vi "Download_All_(Single).vi"(7 "File Selection":i32, 8 "error in (no error)":errorcluster, 10 "Data":T1={"Info Box"="", "MAC & Name Out"=[], "Default Gateway"="", "Drfiter IP Addresses"=[], "Network Map"="", "Drifter Selection"=0, "File Selection"=0, "Download File Path"=path "", "File Selection Strings"=[], "Sample Rate"=enum." 0.2", "Log While Charging"=enum." Yes"}, 11 "File Path Control":path) -> (0 "error out":errorcluster)   [LabVIEW 2017]
uses:
  data.ctl
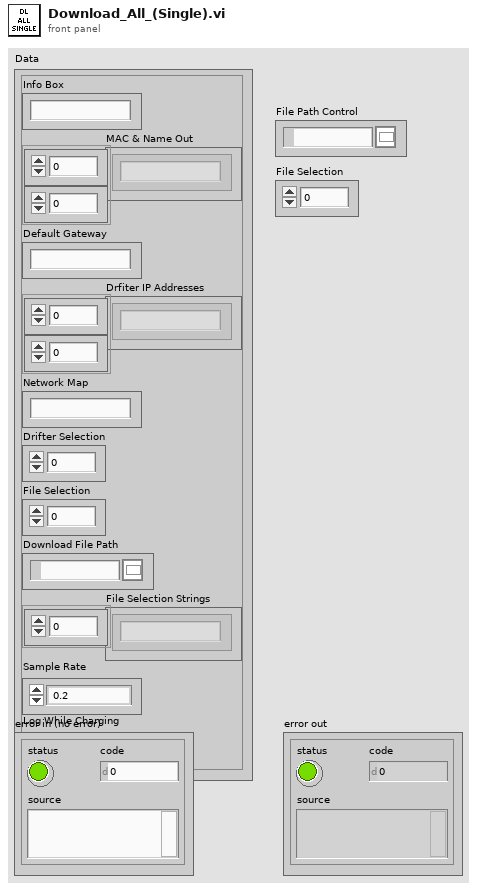
[diagram p1: front panel]
types:
  T1 = typedef "data.ctl" = cluster{"Info Box":string, "MAC & Name Out":string[][], "Default Gateway":string, "Drfiter IP Addresses":string[][], "Network Map":string, "Drifter Selection":i32, "File Selection":i32, "Download File Path":path, "File Selection Strings":string[], "Sample Rate":enum32{"No Selection", " 0.2", " 0.1", " 1", " 2", " 5", " 10"}, "Log While Charging":enum32{"No Selection", " Yes", " No"}}
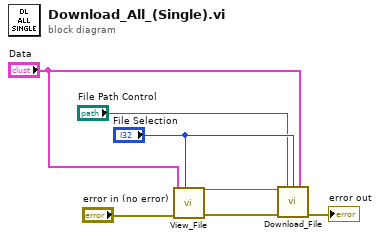
[diagram p0: block diagram]
diagram:
  n1 = call "View_File.vi"("File Selection"="File Selection", "Error In"="error in (no error)", "Data"="Data") -> ("Error Out"=w4:errorcluster, "File Contents"=w2:string)  [unwired: 7 in]
  n2 = call "Download_File.vi"("File Contents"=w2, "File Path Control"="File Path Control", "File Selection"="File Selection", "Data"="Data", "Error In"=w4) -> ("Error Out"=→"error out":errorcluster)  [unwired: 10 in]
